vi "analyseRobotPath.vi"(10 "RRTRobot in":refnum<class "Robot.lvclass">, 11 "OffensiveRobot in":refnum<class "Robot.lvclass">) -> (3 "Robot out":refnum<class "Robot.lvclass">)   [LabVIEW 2023, in "Game.lvclass"]
uses:
  Game.lvclass
  Robot_class/Robot.lvclass
  Robot_class/Robot.lvclass/Robot.ctl
  Robot_class/Read path.vi
  Robot_class/Read path_smooth.vi
  Robot_class/Write path.vi
  Robot_class/Write path_smooth.vi
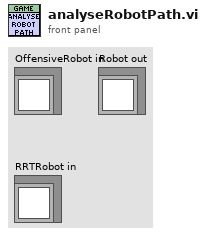
[diagram p1: front panel]
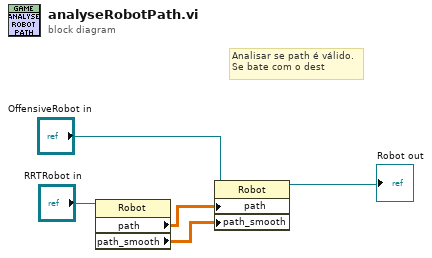
[diagram p0: block diagram]
diagram:
  # "Analisar se path é válido.\nSe bate com o dest"
  n1 = property class="Robot"(reference="RRTRobot in") -> ("path"=w4:dbl[][], "path_smooth"=w5:dbl[][])  [unwired: 1 in, 2 out]
  n2 = property class="Robot"(reference="OffensiveRobot in", "path"=w4, "path_smooth"=w5) -> (reference out=→"Robot out":refnum<class "Robot.lvclass">)  [unwired: 1 in, 1 out]
